vi "Filter Centers.vi"(9 "Center":cluster{"X":dbl, "Y":dbl} {"Y" format="%0.2f"; "X" format="%0.2f"}, 10 "First time":bool, 11 "Centers":cluster{"X":dbl, "Y":dbl}[](array[cluster])) -> (1 "Added":bool, 2 "First time Out":bool, 3 "Centers 2":cluster{"X":dbl, "Y":dbl}[](array[cluster]))   [LabVIEW 2023]
panel:
  out "Y Min":dbl
  out "Y Max":dbl
  out "X Min":dbl
  out "X Max":dbl
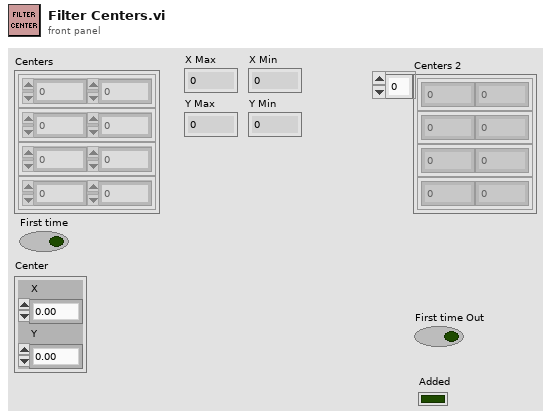
[diagram p1: front panel]
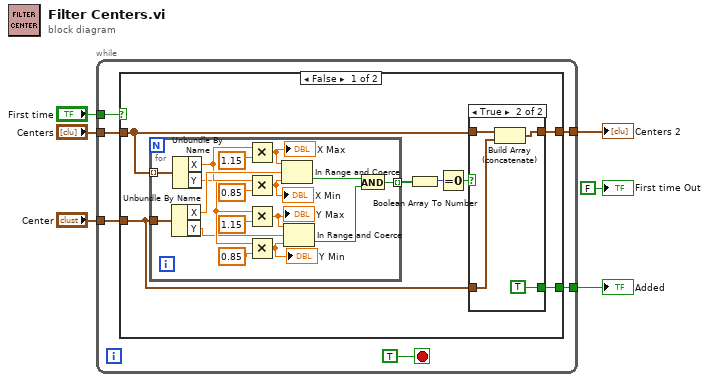
[diagram p0: block diagram]
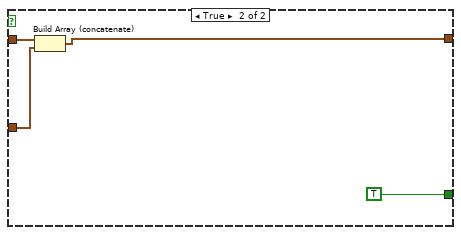
[diagram p3: hidden frame]
diagram:
  n1 = while {
    tunnel: "Centers" -> [w11]
    tunnel: "Center" -> [w12]
    tunnel: [w9] -> w4
    tunnel: [w8] -> w3
    tunnel: "First time" -> [w7]
    stop <- TRUE stop-if-true
    n2 = case shown="False" w7 {
      tunnel: w12 -> [w19 w44]
      tunnel: w11 -> [w18 w45]
      tunnel: [w17 w43] -> w9
      tunnel: [w14 TRUE] -> w8
      frame False {
        n3 = for {
          tunnel: w18 -> [w36] mode=indexing
          tunnel: w19 -> [w22]
          tunnel: [w20] -> w16 mode=indexing
          n4 = Unbundle By Name(w22) -> ("X"=w35:dbl, "Y"=w25:dbl)
          n5 = Unbundle By Name(w36) -> ("X"=w34:dbl, "Y"=w26:dbl)
          n6 = Multiply(x=w34, y=1.15) -> (x*y=w33:dbl)
          "X Max" <- w33
          n7 = Multiply(x=w34, y=0.85) -> (x*y=w31:dbl)
          "X Min" <- w31
          n8 = Multiply(x=w26, y=1.15) -> (x*y=w27:dbl)
          "Y Max" <- w27
          n9 = Multiply(x=w26, y=0.85) -> (x*y=w21:dbl)
          "Y Min" <- w21
          n10 = In Range and Coerce(upper limit=w33, x=w35, lower limit=w31) -> (In Range?=w24:bool)  [unwired: 1 out]
          n11 = In Range and Coerce(upper limit=w27, x=w25, lower limit=w21) -> (In Range?=w23:bool)  [unwired: 1 out]
          n12 = And(x=w24, y=w23) -> (x .and. y?=w20:bool)
        }
        n13 = Boolean Array To Number(Boolean array=w16) -> (number=w15:u32)
        n14 = Equal To 0?(x=w15) -> (x = 0?=w13:bool)
        n15 = case shown="True" w13 {
          tunnel: [w37 w40] -> w17
          tunnel: w18 -> [w37 w41]
          tunnel: w19 -> [_ w39]
          tunnel: [_ TRUE] -> w14
          frame False {
          }
          frame True {
            n16 = Build Array (concatenate)(w41, w39) -> (w40:cluster{"X":dbl, "Y":dbl}[])
          }
        }
      }
      frame True {
        n17 = Build Array (concatenate)(w45, w44) -> (w43:cluster{"X":dbl, "Y":dbl}[])
      }
    }
  }
  "Centers 2" <- w4
  "Added" <- w3
  "First time Out" <- FALSE ("First time Out")
